vi "Create AFDX MAC (Source).vi"(11 "Source Info":T1={"domainID"=0, "sideID"=0, "locationID"=0, "interfaceID"=1} {"interfaceID" format="%.0b"}) -> (3 "MAC-src":u8[](array[numeric]) format="%02x")   [LabVIEW 2020, in "EthFrameManagement.lvlib"]
doc: "Create MAC source from Source Info."
uses:
  EthFrameManagement.lvlib
  controls/mac_src_info_afdx.ctl
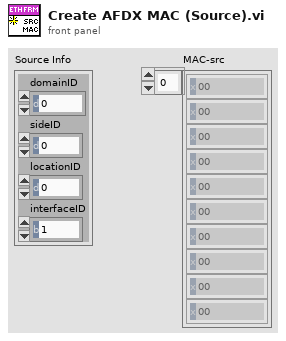
[diagram p1: front panel]
types:
  T1 = typedef "EthFrameManagement.lvlib/mac_src_info_afdx.ctl" = cluster{"domainID":u8, "sideID":u8, "locationID":u8, "interfaceID":u8}
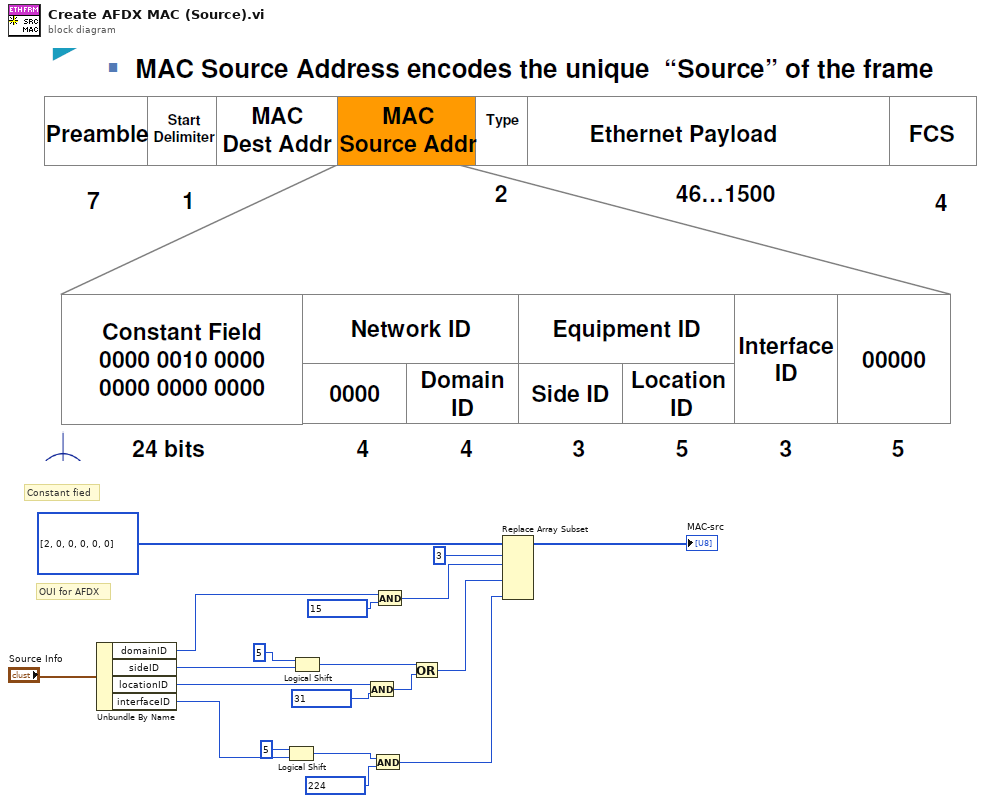
[diagram p0: block diagram]
diagram:
  # "OUI for AFDX"
  # "Constant fied"
  n1 = Unbundle By Name("Source Info") -> ("domainID"=w16:u8, "sideID"=w8:u8, "locationID"=w5:u8, "interfaceID"=w11:u8)
  n2 = Logical Shift(y=i16 5, x=w11) -> (x << y=w9:u8)
  n3 = Logical Shift(y=i16 5, x=w8) -> (x << y=w4:u8)
  n4 = And(x=w5, y=u8 31) -> (x .and. y?=w3:u8)
  n5 = And(x=w9, y=u8 224) -> (x .and. y?=w1:u8)
  n6 = And(x=w16, y=u8 15) -> (x .and. y?=w13:u8)
  n7 = Or(x=w4, y=w3) -> (x .or. y?=w2:u8)
  n8 = Replace Array Subset(array=u8[] [2, 0, 0, 0, 0, 0] ("MAC-src"), new element #1=w13, index #1=3 ("index"), new element #2=w2, new element #3=w1) -> (→"MAC-src":u8[])  [unwired: 2 in]
